vi "CRYLogin Read Config.vi"() -> (0 "Remember Out":bool, 1 "Password out":T1, 2 "Level Out":i32, 3 "Login Section Out":cluster{"Key":string, "Value":string}[](array[cluster]))   [LabVIEW 2013]
panel:
  # "CRYSoundLab Login Read"
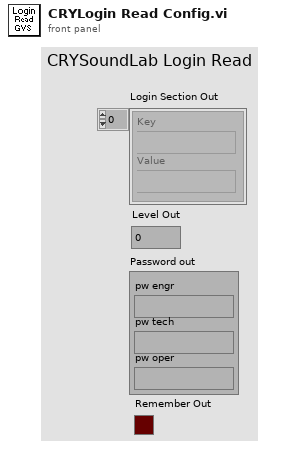
[diagram p1: front panel]
types:
  T1 = cluster{"pw engr":string, "pw tech":string, "pw oper":string}
  T2 = cluster{"Section":string, "Items":cluster{"Key":string, "Value":string}[]}[]
  T3 = cluster{"Section":string, "Items":cluster{"Key":string, "Value":string}[]}
  T4 = cluster{"Value":string, "Value":string, "Value":string}
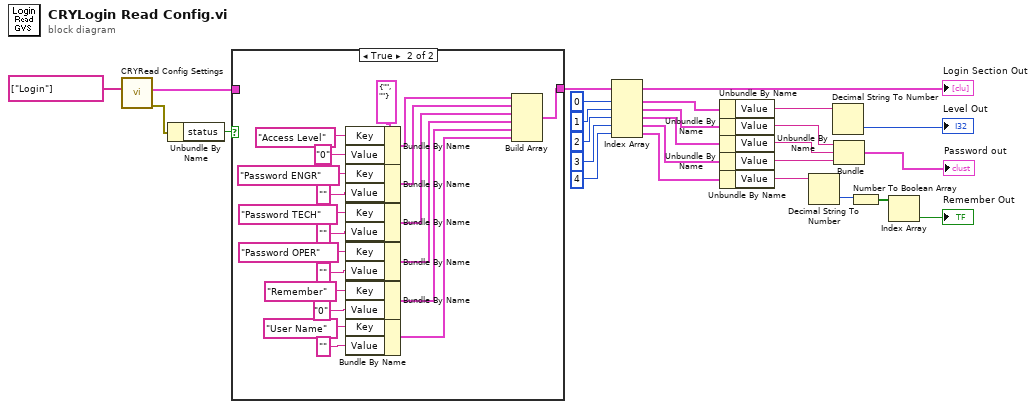
[diagram p0: block diagram]
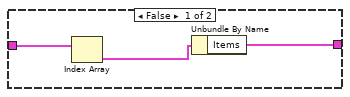
[diagram p2: hidden frame]
diagram:
  n1 = call "CRYRead Config Settings.vi"("Section"=string[] ["Login"]) -> ("error out"=w13:errorcluster, "Configuration Data"=w25:T2)  [unwired: 1 in, 8 out]
  n2 = Unbundle By Name(w13) -> ("status"=w5:bool)
  n3 = case shown="True" w5 {
    tunnel: w25 -> [w27 _]
    tunnel: [w28 w29] -> w2
    frame False {
      n4 = Index Array(array=w27) -> (element=w26:T3)  [unwired: 1 in]
      n5 = Unbundle By Name(w26) -> ("Items"=w28:cluster{"Key":string, "Value":string}[])
    }
    frame True {
      w40 = cluster{"Key":string, "Value":string} {"Key"="", "Value"=""} ("Cluster")
      n6 = Bundle By Name(cluster=w40, "Key"="Access Level", "Value"="0") -> (w43:cluster{"Key":string, "Value":string})
      n7 = Bundle By Name(cluster=w40, "Key"="Password ENGR", "Value"="") -> (w44:cluster{"Key":string, "Value":string})
      n8 = Bundle By Name(cluster=w40, "Key"="Password TECH", "Value"="") -> (w45:cluster{"Key":string, "Value":string})
      n9 = Bundle By Name(cluster=w40, "Key"="Password OPER", "Value"="") -> (w46:cluster{"Key":string, "Value":string})
      n10 = Bundle By Name(cluster=w40, "Key"="Remember", "Value"="0") -> (w47:cluster{"Key":string, "Value":string})
      n11 = Bundle By Name(cluster=w40, "Key"="User Name", "Value"="") -> (w48:cluster{"Key":string, "Value":string})
      n12 = Build Array(w43, w44, w45, w46, w47, w48) -> (w29:cluster{"Key":string, "Value":string}[])
    }
  }
  "Login Section Out" <- w2
  n13 = Index Array(array=w2, index #1=0 ("index"), index #2=1 ("index"), index #3=2 ("index"), index #4=3 ("index"), index #5=4 ("index")) -> (element #1=w24:cluster{"Key":string, "Value":string}, element #2=w16:cluster{"Key":string, "Value":string}, element #3=w4:cluster{"Key":string, "Value":string}, element #4=w15:cluster{"Key":string, "Value":string}, element #5=w14:cluster{"Key":string, "Value":string})
  n14 = Unbundle By Name(w24) -> ("Value"=w23:string)
  n15 = Unbundle By Name(w16) -> ("Value"=w22:string)
  n16 = Unbundle By Name(w4) -> ("Value"=w21:string)
  n17 = Unbundle By Name(w15) -> ("Value"=w20:string)
  n18 = Unbundle By Name(w14) -> ("Value"=w17:string)
  n19 = Decimal String To Number(string=w17) -> (number=w18:i32)  [unwired: 3 out]
  n20 = Decimal String To Number(string=w23) -> (number=→"Level Out":i32)  [unwired: 3 out]
  n21 = Bundle("Value"=w22, "Value"=w21, "Value"=w20) -> (→"Password out":T4)  [unwired: 1 out]
  n22 = Number To Boolean Array(number=w18) -> (Boolean array=w19:bool[])
  n23 = Index Array(array=w19) -> (element=→"Remember Out":bool)  [unwired: 1 in]
